vi "SettingsVI_RUN.vi"(8 "error in (no error)":errorcluster, 10 "user event":refnum<user-event>, 11 "Config in":refnum<class "Config.lvclass">) -> (0 "error out":errorcluster, 3 "reference out":refnum<vi>)   [LabVIEW 2020]
uses:
  Classes/Config/Config.lvclass
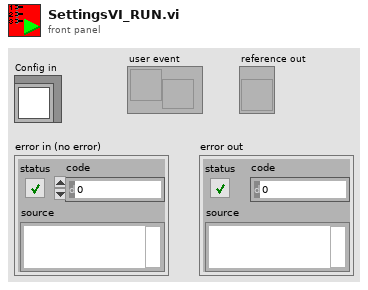
[diagram p1: front panel]
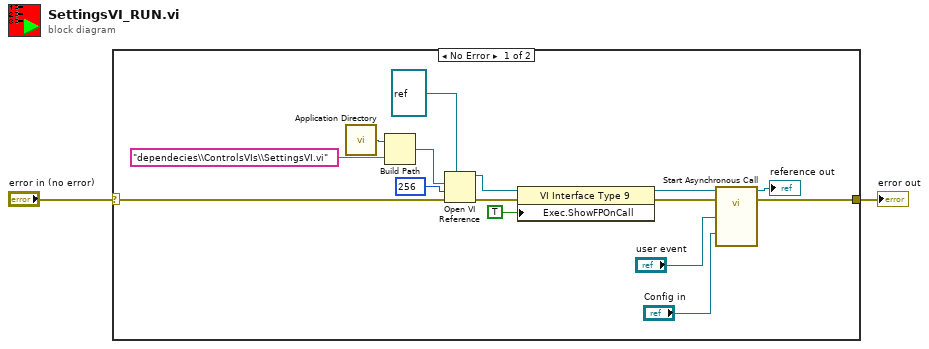
[diagram p0: block diagram]
diagram:
  n1 = case shown="No Error" "error in (no error)" {
    selector: "error in (no error)" -> [w3 w18]
    tunnel: [w8 w18] -> w2
    frame No Error {
      n2 = call <vilib>:"Application Directory.vi"() -> ("Application Directory"=w15:path)
      n3 = Build Path(base path=w15, name or relative path="dependecies\\ControlsVIs\\SettingsVI.vi") -> (appended path=w17:path)
      n4 = Open VI Reference(type specifier VI Refnum (for type only)=refnum<vi> refnum ("spécificateur de type du refnum de VI (pour type seulement)"), vi path=w17, options=256, error in (no error)=w3) -> (vi reference=w12:refnum<vi>, error out=w11:errorcluster)  [unwired: 2 in]
      n5 = property class="VI Interface Type 9"(reference=w12, error in=w11, "Exec.ShowFPOnCall"=TRUE ("Execution:Show Front Panel On Call")) -> (reference out=w6:refnum<vi>, error out=w9:errorcluster)
      n6 = call-by-ref "Start Asynchronous Call"(reference=w6, error in=w9, "Config MAIN"="Config in", "user event"="user event") -> (reference out=→"reference out":refnum<vi>, error out=w8:errorcluster)  [unwired: 1 in]
    }
    frame Error {
    }
  }
  "error out" <- w2
